vi "Thumb Stick RGB LED Example.vi"() -> ()   [LabVIEW 2015, in "LabVIEW Interface for Arduino.lvlib"]
doc: "An example that uses an Arduino to capture input from an analog thumb stick which is used to generate colors based on the angle and magnitude of the thumb stick. These colors are displayed on the front panel and sent to an RGB LED . (The RGB LED can easily be replaced with BlinkMs)"
uses:
  <vilib>/LabVIEW Interface for Arduino/LabVIEW Interface for Arduino.lvlib
panel:
  out "Color":u32(colorbox)=1297
  out "Vertical Axis":dbl(slide)=2.3226 scale=0.0..5.0
  out "Horizontal Axis":dbl(slide)=2.3863 scale=0.0..5.0
  in  "Stop":bool
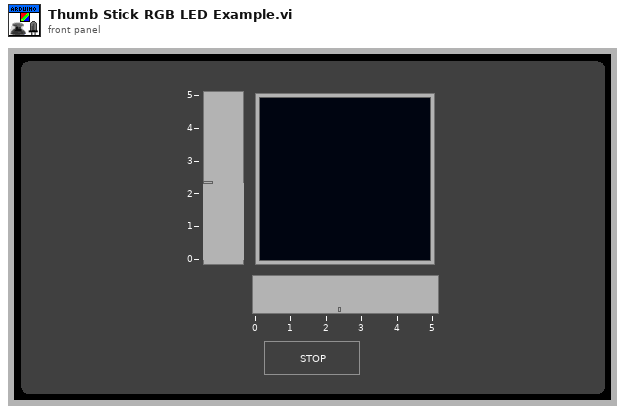
[diagram p1: front panel]
types:
  T1 = typedef "LabVIEW Interface for Arduino.lvlib/Arduino Resource.ctl" = cluster{"VISA resource":refnum<visa-resource-name>, "Board Type":T2, "Connection Type":enum8{"USB / Serial"}, "Bytes Per Packet (15)":u8}
  T2 = typedef "LabVIEW Interface for Arduino.lvlib/Board Type.ctl" = enum16{"Uno", "Dimuelanove w/Atmega 328", "Mega 2560"}
  T3 = cluster{"Horizontal Axis Pin":dbl, "Vertical Axis Pin":dbl, "Select Pin":dbl}
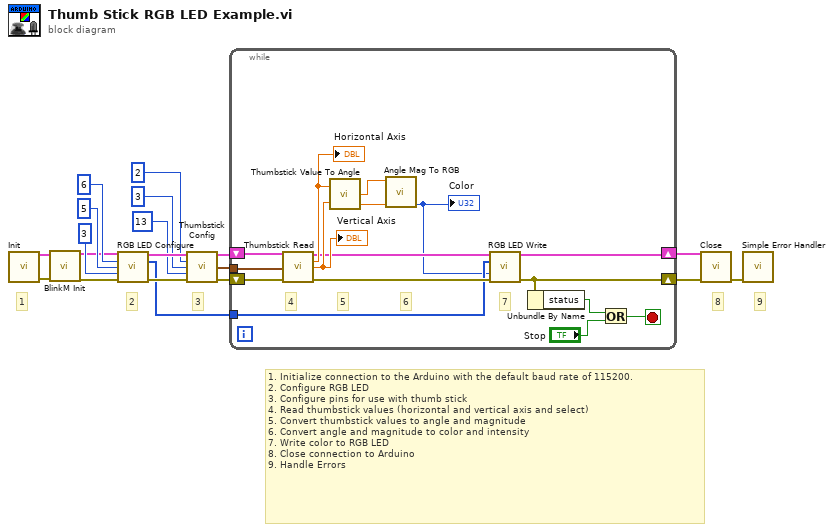
[diagram p0: block diagram]
diagram:
  # "9"
  # "8"
  # "3"
  # "2"
  # "1"
  # "1. Initialize connection to the Arduino with the default baud rate of 115200.\n2. Configure RGB LED\n3. Configure pins for use with thumb stick\n4. Read thumbstick values (horizontal and vertical axis and select)\n5. Convert thumbstick values to angle and magnitude\n6. Convert angle and magnitude to color and intensity\n7. Write color to RGB LED\n8. Close connection to Arduino\n9. Handle Errors"
  n1 = call <vilib>:"Init.vi"() -> ("Arduino Resource"=w4:T1, "error out"=w1:errorcluster)  [unwired: 18 in]
  n2 = call <vilib>:"BlinkM Init.vi"("Arduino Resource"=w4, "error in"=w1) -> ("Arduino Resource"=w3:T1, "error out"=w2:errorcluster)  [unwired: 12 in]
  n3 = call <vilib>:"RGB LED Configure.vi"("Arduino Resource"=w3, "Red Pin"=u8 6, "Green Pin"=u8 5, "Blue Pin"=u8 3, "error in"=w2) -> ("Arduino Resource"=w14:T1, "RGB LED Pins"=w5:u8[], "error out"=w13:errorcluster)  [unwired: 8 in]
  n4 = call <vilib>:"Thumbstick Config.vi"("Arduino Resource"=w14, "Horizontal Axis AI Pin"=u8 2, "Vertical Axis AI Pin"=u8 3, "Select DI Pin"=u8 13, "error in"=w13) -> ("Arduino Resource"=w18:T1, "Thumbstick Data"=w19:T3, "error out"=w17:errorcluster)  [unwired: 8 in]
  n5 = while {
    shift-right: [w21] -> w7
    shift-left: w18 -> [w35]
    shift-right: [w20] -> w16
    shift-left: w17 -> [w34]
    tunnel: w19 -> [w33]
    tunnel: w5 -> [w23]
    stop <- w25 stop-if-true
    # "7"
    # "6"
    # "5"
    # "4"
    n6 = call <vilib>:"Thumbstick Read.vi"("Arduino Resource"=w35, "Thumbstick Data"=w33, "error in"=w34) -> ("Arduino Resource"=w24:T1, "Horizontal Axis"=w30:dbl, "Vertical Axis"=w29:dbl, "error out"=w28:errorcluster)  [unwired: 8 in, 1 out]
    "Horizontal Axis" <- w30
    "Vertical Axis" <- w29
    n7 = call <vilib>:"Thumbstick Value To Angle.vi"("Vertical Axis"=w29, "Horizontal Axis"=w30) -> ("Magnitude"=w32:dbl, "Degrees"=w31:dbl)  [unwired: 1 out]
    n8 = call <vilib>:"Angle Mag To RGB.vi"("Magnitude (0-1)"=w32, "Angle (Degrees)"=w31) -> ("RGB Color"=w22:u32)  [unwired: 6 in, 3 out]
    "Color" <- w22
    n9 = call <vilib>:"RGB LED Write.vi"("Arduino Resource"=w24, "RGB LED Pins"=w23, "Color"=w22, "error in"=w28) -> ("Arduino Resource"=w21:T1, "error out"=w20:errorcluster)  [unwired: 9 in, 1 out]
    n10 = Unbundle By Name(w20) -> ("status"=w27:bool)
    n11 = Or(x=w27, y="Stop") -> (x .or. y?=w25:bool)
  }
  n12 = call <vilib>:"Close.vi"("Arduino Resource"=w7, "error in"=w16) -> ("error out"=w15:errorcluster)  [unwired: 13 in]
  n13 = call <vilib>:"Simple Error Handler.vi"("error in (no error)"=w15) -> ()  [unwired: 4 in, 5 out]
